vi "find_daq.vi"(0 "Device Name":string="USB-6008") -> (1 "Device Present":bool, 2 "DAQmx Device Name":tag)   [LabVIEW 2013]
doc: "This VI takes a device type input (ex. PCI-6251, USB-6008, etc.) and returns the resource name specified in Measurement and Automation Explorer."
uses:
  <resource>/objmgr/daqmx.rc
panel:
  out "DevSerialNum":u32
  # "Input"
  # "Output"
  # "Input the Desired DAQ device \nto be used in your program"
  # "This is the Device Name that is set in MAX.  This name \nrepresents the resource input for your Task."
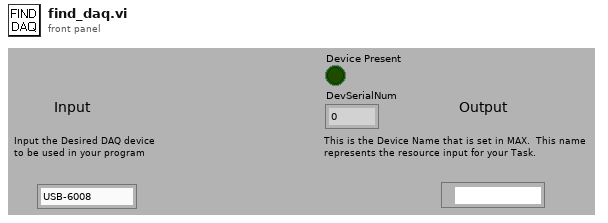
[diagram p1: front panel]
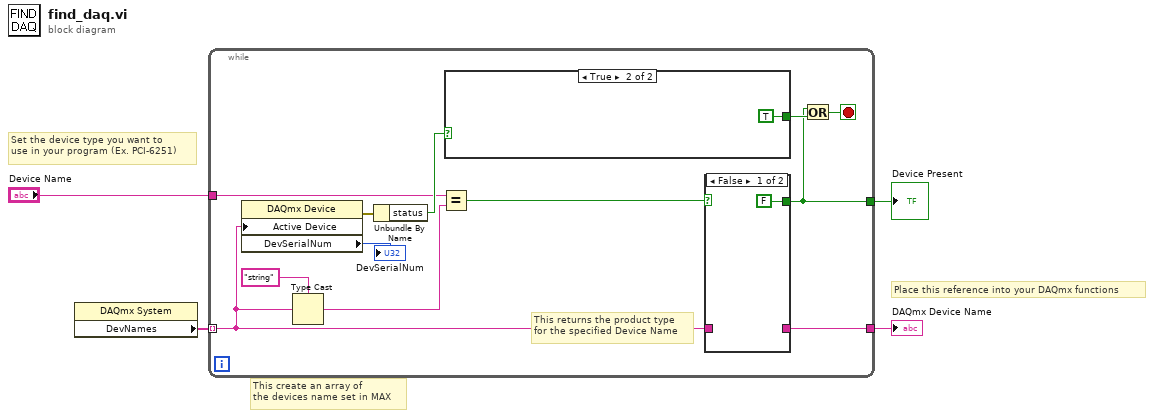
[diagram p0: block diagram]
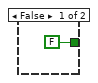
[diagram p2: hidden frame]
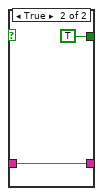
[diagram p3: hidden frame]
diagram:
  # "Place this reference into your DAQmx functions"
  # "Set the device type you want to \nuse in your program (Ex. PCI-6251)"
  # "This create an array of \nthe devices name set in MAX"
  n1 = property class="DAQmx System"() -> ("DevNames"=w3:tag[])  [unwired: 2 in, 2 out]
  n2 = while {
    tunnel: w3 -> [w9] mode=indexing
    tunnel: [w14] -> w2
    tunnel: "Device Name" -> [w6]
    tunnel: [w10] -> w1
    stop <- w16 stop-if-true
    # "This returns the product type\nfor the specified Device Name"
    n3 = property class="DAQmx Device"("Active Device"=w9) -> (error out=w13:errorcluster, "DevSerialNum"=→"DevSerialNum":u32)  [unwired: 2 in, 1 out]
    n4 = Type Cast(type="string", x=w9) -> (*(type *) &x=w7:string)
    n5 = Unbundle By Name(w13) -> ("status"=w12:bool)
    n6 = Equal?(x=w6, y=w7) -> (x = y?=w15:bool)
    n7 = case shown="True" w12 {
      tunnel: [FALSE ("true") TRUE ("true")] -> w11
      frame False {
      }
      frame True {
      }
    }
    n8 = case shown="False" w15 {
      tunnel: [_ w21] -> w14
      tunnel: w9 -> [_ w21]
      tunnel: [FALSE TRUE] -> w10
      frame False {
      }
      frame True {
      }
    }
    n9 = Or(x=w10, y=w11) -> (x .or. y?=w16:bool)
  }
  "DAQmx Device Name" <- w2
  "Device Present" <- w1
